vi "MPPT.vi"() -> ()   [LabVIEW 2017]
doc: "This example shows how to create, run a script and query the script output data."
uses:
  <instrlib>/Keithley 2600 Series/Keithley 2600 Series.lvlib
panel:
  out "PCE(a.u.)":dbl
  in  "Pin(W/cm^2)":dbl
  out "FF(a.u.)":dbl
  out "Jsc(A/cm^2)":dbl
  in  "Area(cm^2)":dbl
  out "Voc(V)":dbl
  out "Ioc(A)":dbl
  out "Vsc(V)":dbl
  out "Isc(A)":dbl
  out "IMP(A)":dbl
  out "VMP(V)":dbl
  out "PMP(W)":dbl
  out "output array":string[][](array[string])
  in  "SweepSetting":T1={"CurrentLimit(A)"=1e-08, "Start Voltage(V)"=0.0} {"Start Voltage(V)" min=-200.0 max=200.0; "CurrentLimit(A)" min=1e-09 max=1.5}
  out "Graph 2":cluster{"Y":dbl[], "Y":dbl[]}[](graph)
  in  "USB COM Port":refnum<visa-resource-name>
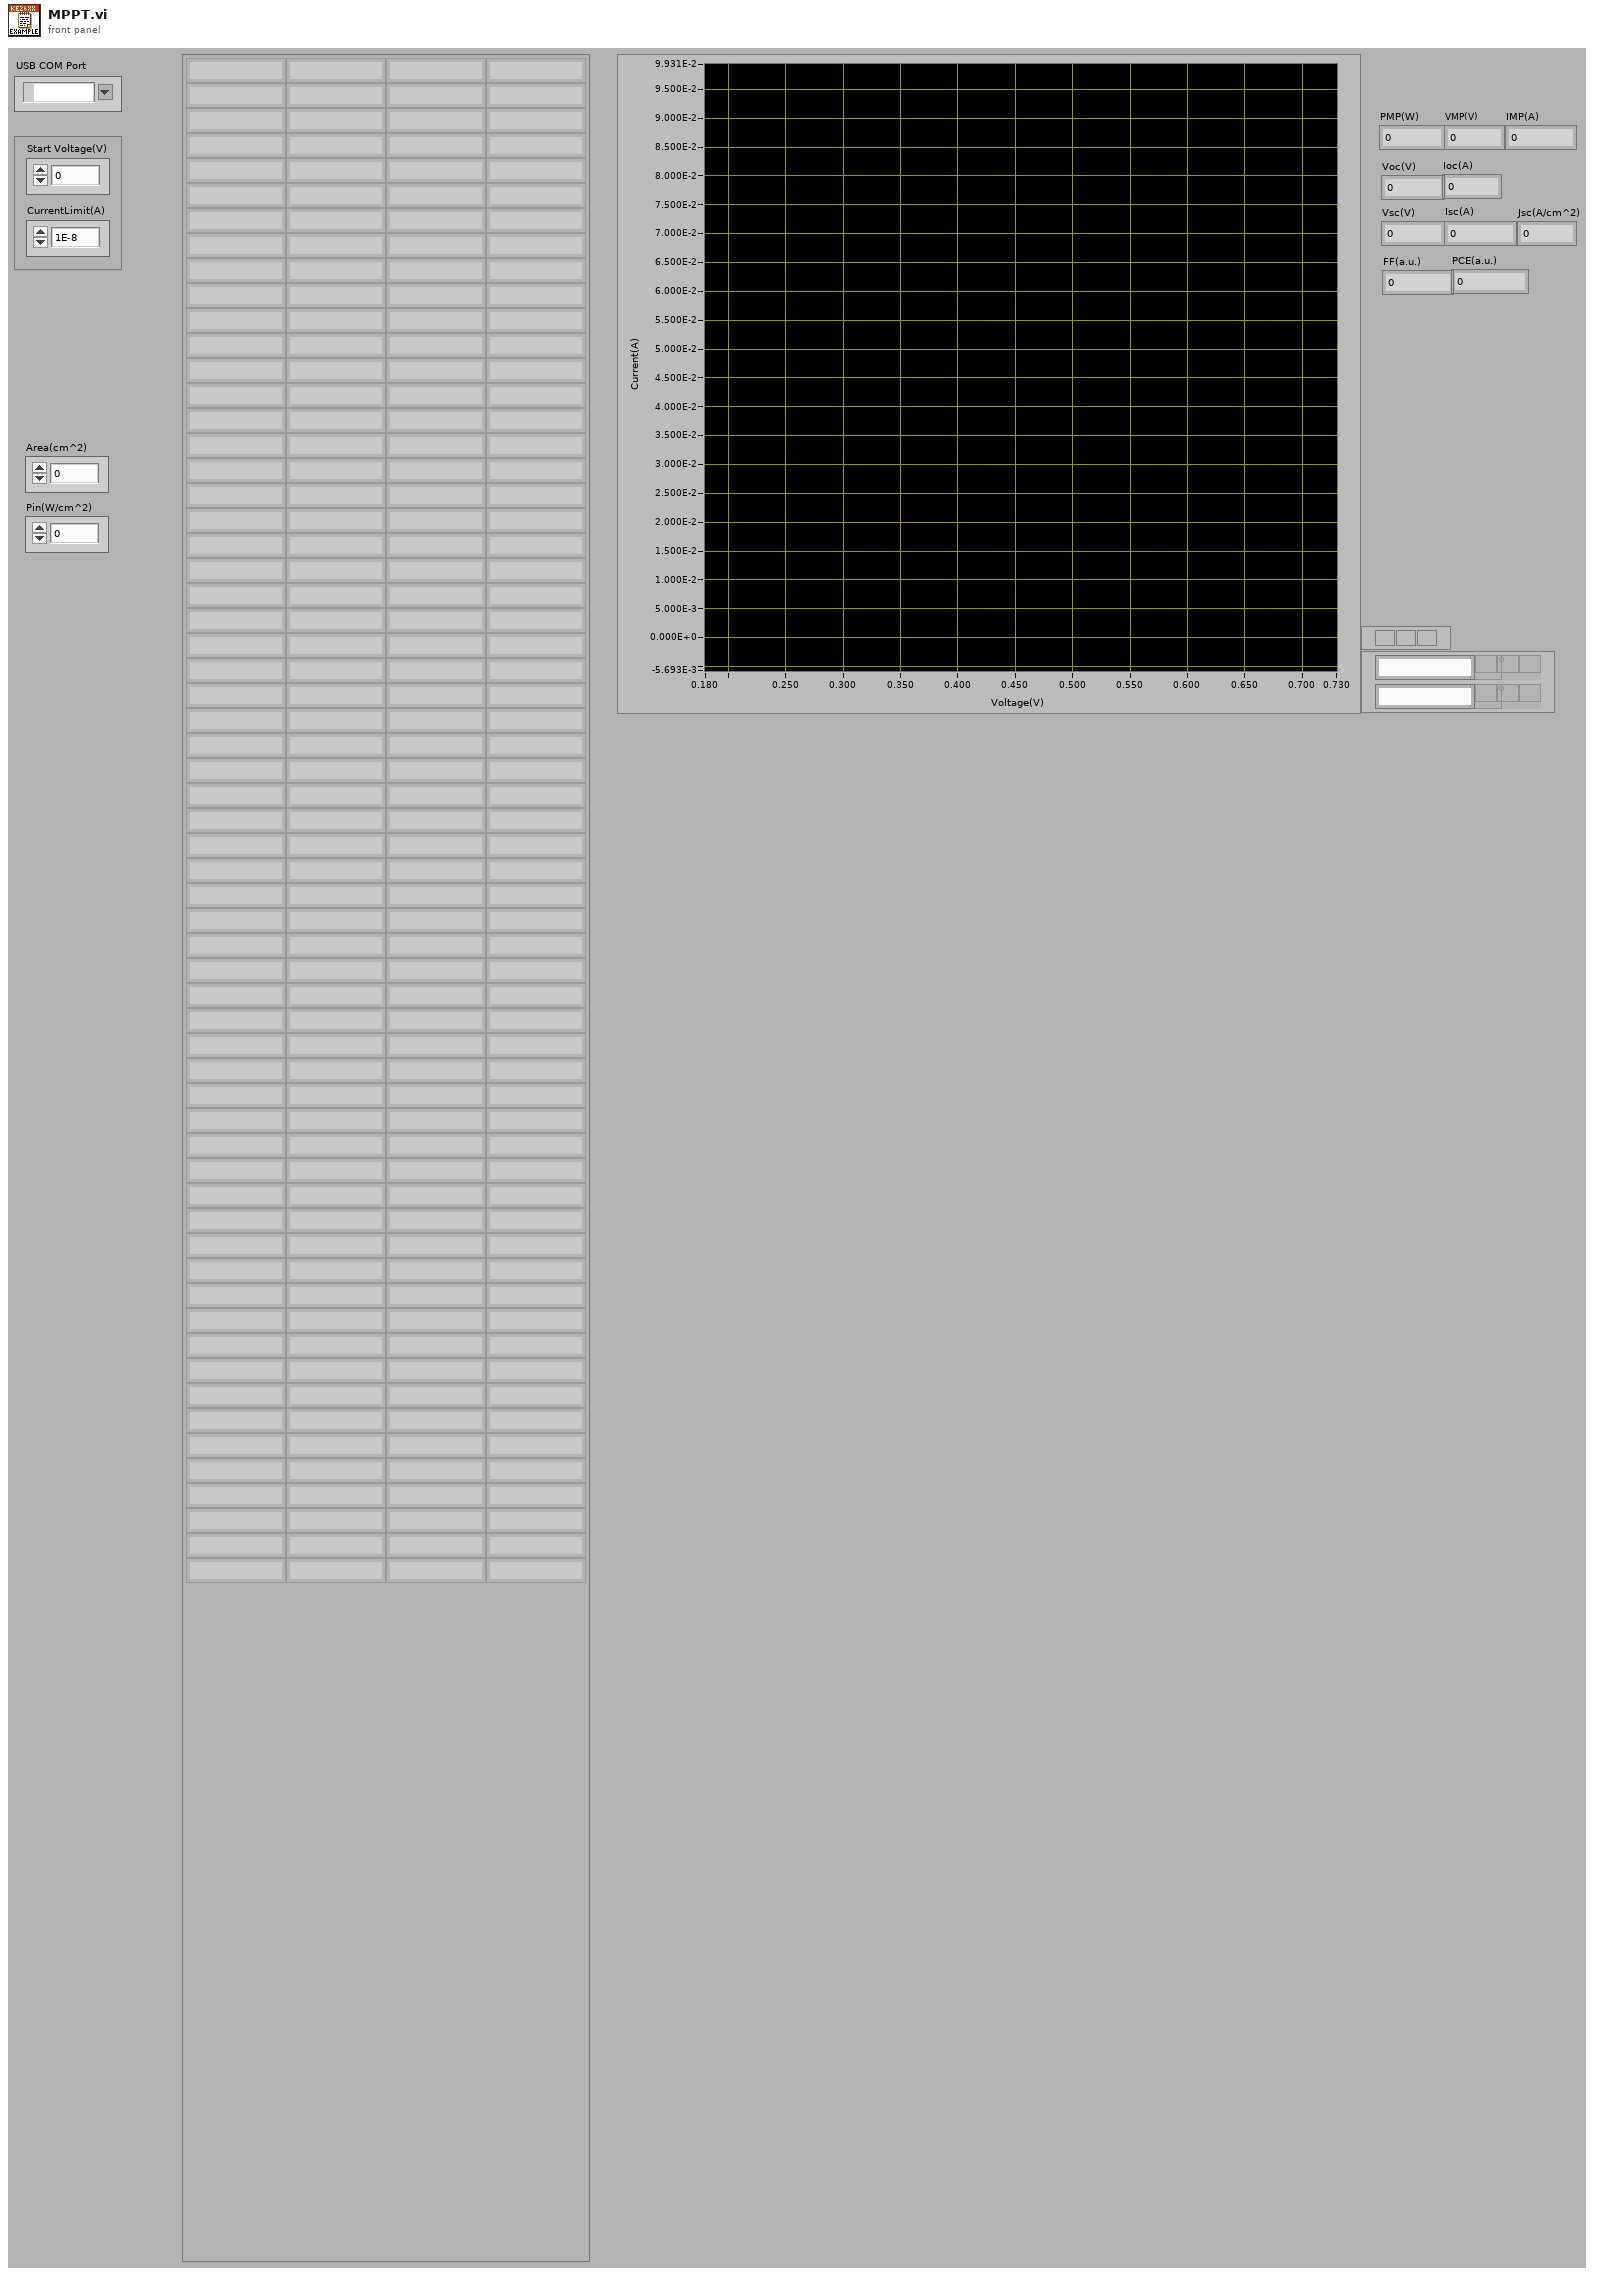
[diagram p1: front panel]
types:
  T1 = cluster{"CurrentLimit(A)":dbl, "Start Voltage(V)":dbl}
  T2 = cluster{"Baud Rate":u32, "Parity":u16, "Data Bits":u16, "Stop Bits":u16, "Flow Control":u16}
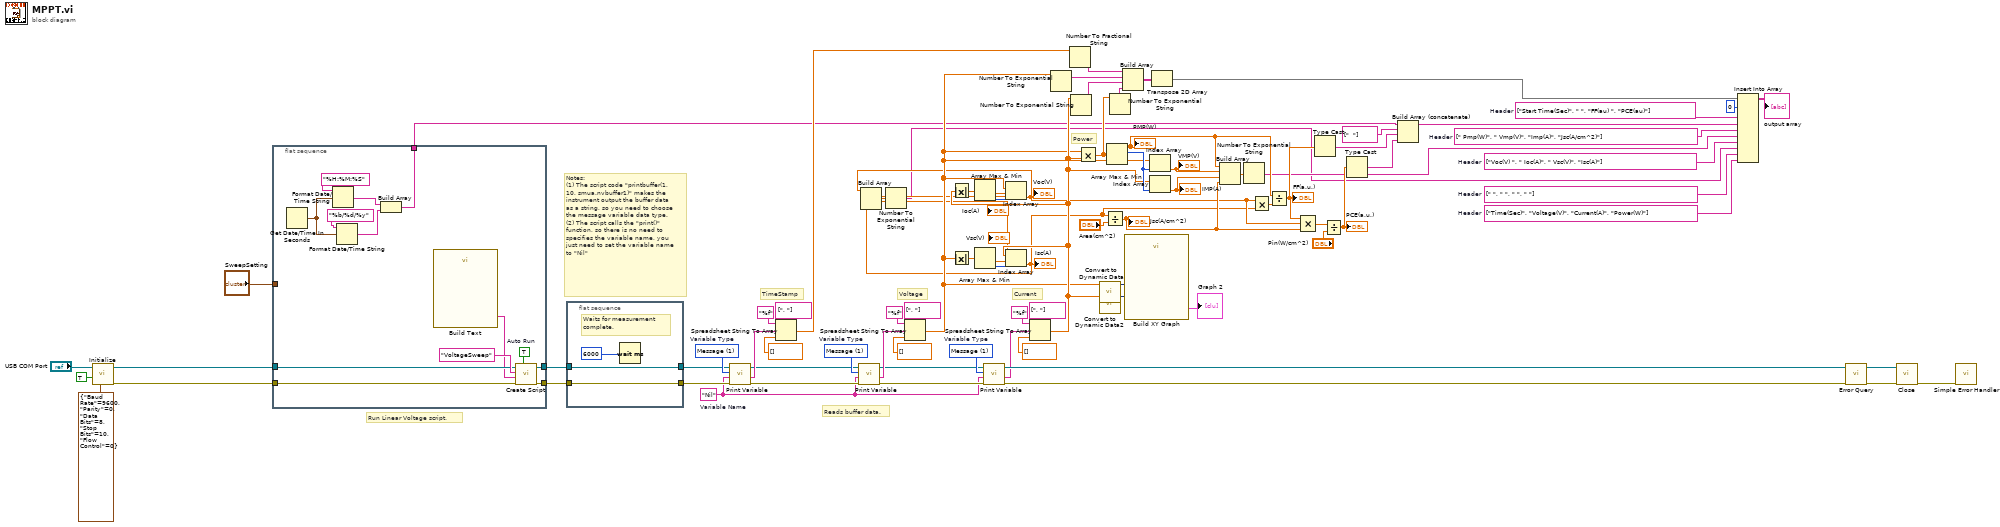
[diagram p0: block diagram]
diagram:
  w4 = string[] ["Voc(V) ", " Ioc(A)", " Vsc(V)", "Isc(A)"]  # Header
  w5 = string[] [" Pmp(W)", " Vmp(V)", "Imp(A)", "Jsc(A/cm^2)"]  # Header
  w1 = string[] ["Time(Sec)", "Voltage(V)", "Current(A)", "Power(W)"]  # Header
  w2 = string[] [" ", " ", " ", " "]  # Header
  w18 = string[] ["Start Time(Sec)", " ", "FF(au) ", "PCE(au)"]  # Header
  w59 = 1 items=["Number", "Message"]  # Variable Type
  w60 = 1 items=["Number", "Message"]  # Variable Type
  w82 = 1 items=["Number", "Message"]  # Variable Type
  w48 = "Nil"  # Variable Name
  # "Power"
  # "Current"
  # "Voltage"
  # "TimeStamp"
  # "Reads buffer data."
  # "Notes: \n(1) The script code \"printbuffer(1, 10, smua.nvbuffer1)\" makes the instrument output the buffer data as a string, so you need to choose the message variable data type.\n(2) The script calls the \"print()\" function, so there is no need to specifies the variable name, you just need to set the variable name to \"Nil\""
  # "Run Linear Voltage script."
  n1 = call <instrlib>:"Initialize.vi"("Serial Configuration"=T2 {"Baud Rate"=9600, "Parity"=0, "Data Bits"=8, "Stop Bits"=10, "Flow Control"=0}, "Reset (True)"=TRUE, "VISA resource name"="USB COM Port") -> ("error out"=w73:errorcluster, "VISA resource name out"=w74:refnum<visa-resource-name>)  [unwired: 7 in]
  n2 = flat-sequence {
    tunnel: [w95] -> w81
    tunnel: [w94] -> w80
    tunnel: w74 -> [w93]
    tunnel: w73 -> [w92]
    tunnel: "SweepSetting" -> [w90]
    tunnel: [w84] -> w24
    frame #0 {
      w96 = TRUE  # Auto Run
      n3 = Get Date/Time In Seconds() -> (seconds since 1Jan1904=w85:timestamp)
      n4 = Format Date/Time String(time format string (%c)="%H:%M:%S", seconds (now)=w85) -> (date/time string=w88:string)  [unwired: 1 out]
      n5 = Format Date/Time String(time format string (%c)="%b/%d/%y", seconds (now)=w85) -> (date/time string=w86:string)  [unwired: 1 out]
      n6 = Build Array(w88, w86) -> (w84:string[])
      n7 = call "Build Text"() -> ("Result"=w91:string)  [unwired: 14 in, 1 out]
      n8 = call <instrlib>:"Create Script.vi"("Auto Run (F: Disable)"=w96, "error in (no error)"=w92, "Source Code"=w91, "Script Variable"="VoltageSweep" ("Script Variable (myScript)"), "VISA resource name"=w93) -> ("error out"=w94:errorcluster, "VISA resource name out"=w95:refnum<visa-resource-name>)  [unwired: 5 in]
    }
  }
  n9 = flat-sequence {
    tunnel: w81 -> [w98]
    tunnel: w80 -> [w99]
    tunnel: [w99] -> w78
    tunnel: [w98] -> w79
    frame #0 {
      # "Waits for measurement complete."
      n10 = Wait (ms)(milliseconds to wait=6000 ("Temp Delay")) -> ()  [unwired: 1 out]
    }
  }
  n11 = call <instrlib>:"Print Variable.vi"("error in (no error)"=w78, "Variable Name"=w48, "Variable Type (0: Number)"=w82, "VISA resource name"=w79) -> ("error out"=w56:errorcluster, "Message"=w65:string, "VISA resource name out"=w57:refnum<visa-resource-name>)  [unwired: 4 in, 1 out]
  n12 = Spreadsheet String To Array(delimiter (Tab)=string[] [", "], format string="%f", spreadsheet string=w65, array type (2D Dbl)=dbl[] []) -> (array=w42:dbl[])
  n13 = call <instrlib>:"Print Variable.vi"("error in (no error)"=w56, "Variable Name"=w48, "Variable Type (0: Number)"=w60, "VISA resource name"=w57) -> ("error out"=w54:errorcluster, "Message"=w64:string, "VISA resource name out"=w55:refnum<visa-resource-name>)  [unwired: 4 in, 1 out]
  n14 = Spreadsheet String To Array(delimiter (Tab)=string[] [", "], format string="%f", spreadsheet string=w64, array type (2D Dbl)=dbl[] []) -> (array=w31:dbl[])
  n15 = Absolute Value(x=w31) -> (abs(x)=w36:dbl[])
  n16 = Array Max & Min(array=w36) -> (min value=w7:dbl, min index (indices)=w35:i32)  [unwired: 2 out]
  "Vsc(V)" <- w7
  n17 = call <instrlib>:"Print Variable.vi"("error in (no error)"=w54, "Variable Name"=w48, "Variable Type (0: Number)"=w59, "VISA resource name"=w55) -> ("error out"=w52:errorcluster, "Message"=w50:string, "VISA resource name out"=w53:refnum<visa-resource-name>)  [unwired: 4 in, 1 out]
  n18 = Spreadsheet String To Array(delimiter (Tab)=string[] [", "], format string="%f", spreadsheet string=w50, array type (2D Dbl)=dbl[] []) -> (array=w32:dbl[])
  n19 = Absolute Value(x=w32) -> (abs(x)=w33:dbl[])
  n20 = Array Max & Min(array=w33) -> (min value=w8:dbl, min index (indices)=w34:i32)  [unwired: 2 out]
  "Ioc(A)" <- w8
  n21 = Index Array(array=w31, index=w34) -> (element=w9:dbl)
  "Voc(V)" <- w9
  n22 = Index Array(array=w32, index=w35) -> (element=w6:dbl)
  "Isc(A)" <- w6
  n23 = Build Array(w9, w8, w7, w6) -> (w10:dbl[])
  n24 = Number To Exponential String(number=w10) -> (E-format string=w3:string[])  [unwired: 3 in]
  n25 = Number To Exponential String(number=w31) -> (E-format string=w45:string[])  [unwired: 3 in]
  n26 = Number To Fractional String(number=w42) -> (F-format string=w46:string[])  [unwired: 3 in]
  n27 = Number To Exponential String(number=w32) -> (E-format string=w40:string[])  [unwired: 3 in]
  n28 = Multiply(x=w31, y=w32) -> (x*y=w25:dbl[])
  n29 = call "Convert to Dynamic Data"("Array"=w31) -> ("Dynamic Data Type"=w39:dynamicdata)  [unwired: 3 in]
  n30 = call "Convert to Dynamic Data2"("Array"=w32) -> ("Dynamic Data Type"=w38:dynamicdata)  [unwired: 3 in]
  n31 = Divide(x=w6, y="Area(cm^2)") -> (x/y=w13:dbl)
  "Jsc(A/cm^2)" <- w13
  n32 = Array Max & Min(array=w25) -> (max value=w16:dbl, max index (indices)=w37:i32)  [unwired: 2 out]
  "PMP(W)" <- w16
  n33 = Number To Exponential String(number=w25) -> (E-format string=w26:string[])  [unwired: 3 in]
  n34 = Build Array(w46, w45, w40, w26) -> (w47:string[][])
  n35 = call "Build XY Graph"("Y Input"=w38, "X Input"=w39) -> ("XY Graph"=→"Graph 2":cluster{"X":dbl[], "Y":dbl[]}[])  [unwired: 8 in, 1 out]
  n36 = Index Array(array=w31, index=w37) -> (element=w15:dbl)
  "VMP(V)" <- w15
  n37 = Index Array(array=w32, index=w37) -> (element=w14:dbl)
  "IMP(A)" <- w14
  n38 = Transpose 2D Array(2D array=w47) -> (transposed array=w44:string[][])
  n39 = Build Array(w16, w15, w14, w13) -> (w12:dbl[])
  n40 = Number To Exponential String(number=w12) -> (E-format string=w11:string[])  [unwired: 3 in]
  n41 = Multiply(x=w6, y=w9) -> (x*y=w29:dbl)
  n42 = Divide(x=w16, y=w29) -> (x/y=w22:dbl)
  "FF(a.u.)" <- w22
  n43 = Compound Arithmetic op=MULTIPLY(w22, w9, w13) -> (w28:dbl)
  n44 = Type Cast(x=w22) -> (*(type *) &x=w21:string)  [unwired: 1 in]
  n45 = Divide(x=w28, y="Pin(W/cm^2)") -> (x/y=w19:dbl)
  "PCE(a.u.)" <- w19
  n46 = Type Cast(x=w19) -> (*(type *) &x=w20:string)  [unwired: 1 in]
  n47 = Build Array (concatenate)(w24, string[] ["  "] ("element"), w21, w20) -> (w17:string[])
  n48 = Insert Into Array(array=w44, index (row)=0, new element #1=w18, new element #2=w17, new element #3=w5, new element #4=w11, new element #5=w4, new element #6=w3, new element #7=w2, new element #8=w1) -> (→"output array":string[][])  [unwired: 1 in]
  n49 = call <instrlib>:"Error Query.vi"("error in (no error)"=w52, "VISA resource name"=w53) -> ("error out"=w76:errorcluster, "VISA resource name out"=w77:refnum<visa-resource-name>)  [unwired: 6 in, 2 out]
  n50 = call <instrlib>:"Close.vi"("error in (no error)"=w76, "VISA resource name"=w77) -> ("error out"=w83:errorcluster)  [unwired: 9 in]
  n51 = call <vilib>:"Simple Error Handler.vi"("error in (no error)"=w83) -> ()  [unwired: 4 in, 5 out]
